vi "UDP_send_conditional_v03.vi"() -> ()   [LabVIEW 2025]
uses:
  <vilib>/Utility/file.llb/Write Delimited Spreadsheet (DBL).vi
panel:
  out "Sine 2":dynamicdata(graph) caption="Sine"
  in  "append to file? (new file:F) 2":bool
  in  "append to file? (new file:F)":bool
  in  "stop":bool
  out "Sine":dynamicdata(graph)
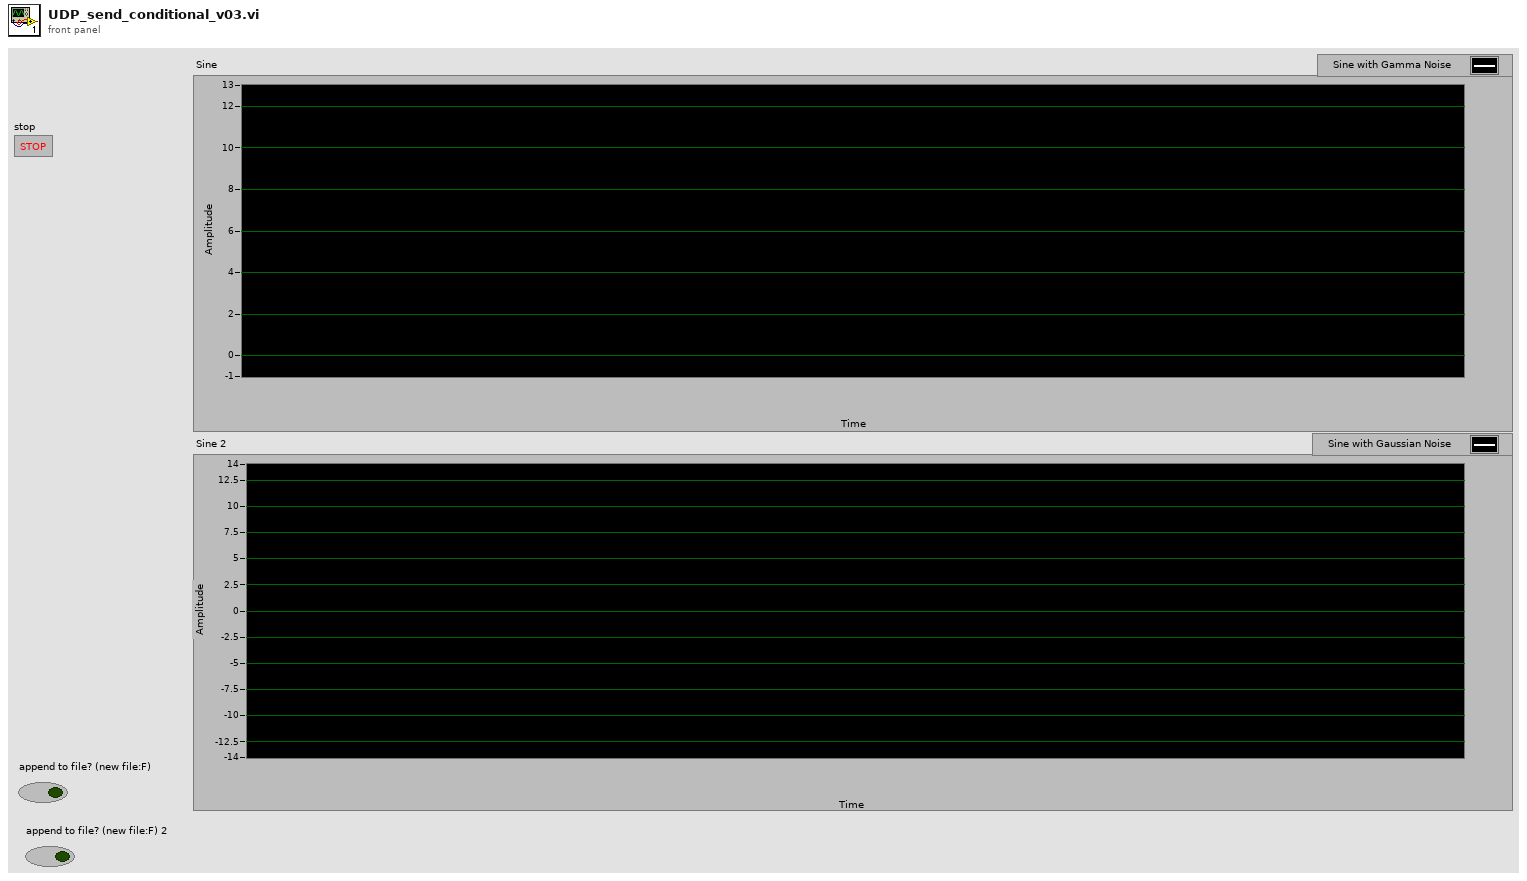
[diagram p1: front panel]
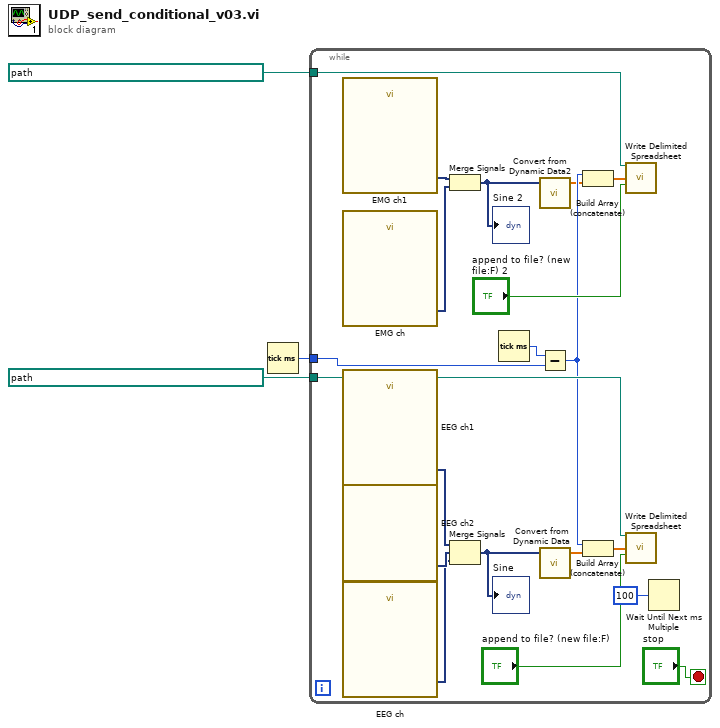
[diagram p0: block diagram]
diagram:
  n1 = Tick Count (ms)() -> (millisecond timer value=w2:u32)
  n2 = while {
    tunnel: path "/home/seidi/Área de trabalho/test_signal1.csv" ("file path (dialog if empty)") -> [w21]
    tunnel: w2 -> [w18]
    tunnel: path "/home/seidi/Área de trabalho/test_signal2.csv" ("file path (dialog if empty)") -> [w15]
    stop <- "stop" stop-if-true
    n3 = call "EMG ch1"() -> ("Sine with Gaussian Noise"=w10:dynamicdata)  [unwired: 14 in, 1 out]
    n4 = call "EMG ch"() -> ("Sine with Gaussian Noise"=w9:dynamicdata)  [unwired: 14 in, 1 out]
    n5 = call "EEG ch1"() -> ("Sine with Gamma Noise"=w6:dynamicdata)  [unwired: 14 in, 1 out]
    n6 = call "EEG ch2"() -> ("Sine with Gamma Noise"=w5:dynamicdata)  [unwired: 14 in, 1 out]
    n7 = call "EEG ch"() -> ("Sine with Gamma Noise"=w4:dynamicdata)  [unwired: 14 in, 1 out]
    n8 = Merge Signals(w10, w9) -> (w8:dynamicdata)
    "Sine 2" <- w8
    n9 = Merge Signals(w6, w5, w4) -> (w22:dynamicdata)
    "Sine" <- w22
    n10 = Tick Count (ms)() -> (millisecond timer value=w17:u32)
    n11 = call "Convert from Dynamic Data2"("Dynamic Data Type"=w8) -> ("Array"=w7:dbl[])  [unwired: 3 in]
    n12 = Subtract(x=w17, y=w18) -> (x-y=w13:u32)
    n13 = call "Convert from Dynamic Data"("Dynamic Data Type"=w22) -> ("Array"=w11:dbl[])  [unwired: 3 in]
    n14 = Build Array (concatenate)(w13, w7) -> (w12:dbl[])
    n15 = Build Array (concatenate)(w13, w11) -> (w19:dbl[])
    n16 = call-poly <vilib>:"Write Delimited Spreadsheet.vi"("file path (dialog if empty)"=w15, "1D data"=w12, "append to file? (new file:F)"="append to file? (new file:F) 2") -> ()  [unwired: 11 in, 2 out]
    n17 = call-poly <vilib>:"Write Delimited Spreadsheet.vi"("file path (dialog if empty)"=w21, "1D data"=w19, "append to file? (new file:F)"="append to file? (new file:F)") -> ()  [unwired: 11 in, 2 out]
    n18 = Wait Until Next ms Multiple(millisecond multiple=u32 100) -> ()  [unwired: 1 out]
  }
